vi "Read Strings from File.vi"(8 "Error In":errorcluster, 9 "Section Name":string, 11 "Path":path) -> (0 "Error Out":errorcluster, 1 "Found?":bool, 3 "Variant Database":variant)   [LabVIEW 2015]
doc: "This VI was created for use with the Read/Write Cluster VIs. It reads all the keys and their values from the specified section and puts them in two string arrays.\n\nFreeware from Moore Good Ideas, www.mooregoodideas.com. Do not remove this line."
uses:
  Suppress Error Code - Scalar.vi
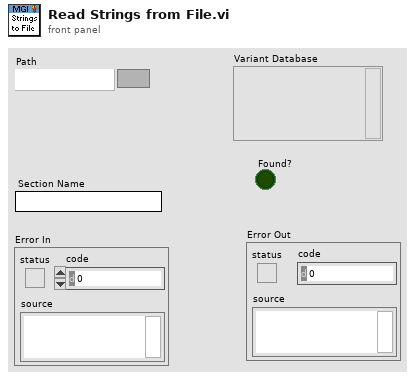
[diagram p1: front panel]
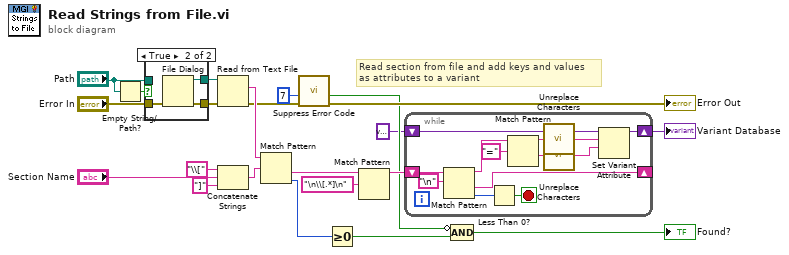
[diagram p0: block diagram]
diagram:
  # "Read section from file and add keys and values\nas attributes to a variant"
  n1 = Empty String/Path?(string/path="Path") -> (empty?=w2:bool)
  n2 = case shown="True" w2 {
    tunnel: "Error In" -> [w23 w27]
    tunnel: [w23 w26] -> w3
    tunnel: [w24 w25] -> w5
    tunnel: "Path" -> [w24 _]
    frame False {
    }
    frame True {
      n3 = File Dialog(8:w27) -> (0:w26:errorcluster, 3:w25:path)  [unwired: 8 out]
    }
  }
  n4 = Read from Text File(file (use dialog)=w5, error in=w3) -> (text=w18:string, error out=w14:errorcluster)  [unwired: 4 out]
  n5 = Concatenate Strings("\\[" ("string"), "Section Name", "]" ("string")) -> (w19:string)
  n6 = Match Pattern(string=w18, regular expression=w19) -> (after substring=w13:string, offset past match=w15:i32)  [unwired: 3 out]
  n7 = call-poly "Suppress Error Code.vi"("Error In"=w14, "Error Code"=7) -> ("Error Out"=→"Error Out":errorcluster, "Error Supressed?"=w9:bool)  [unwired: 8 out]
  n8 = Greater Or Equal To 0?(x=w15) -> (x >= 0?=w10:bool)
  n9 = Match Pattern(string=w13, regular expression="\n\\[.*]\n") -> (before substring=w16:string)  [unwired: 4 out]
  n10 = while {
    shift-right: [w38] -> _
    shift-left: w16 -> [w40]
    shift-right: [w33] -> w6
    shift-left: variant ("variant") -> [w34]
    stop <- w36 stop-if-true
    n11 = Match Pattern(string=w40, regular expression="\n") -> (before substring=w32:string, after substring=w38:string, offset past match=w37:i32)  [unwired: 2 out]
    n12 = Less Than 0?(x=w37) -> (x < 0?=w36:bool)
    n13 = Match Pattern(string=w32, regular expression="=") -> (before substring=w31:string, after substring=w30:string)  [unwired: 3 out]
    n14 = call "Unreplace Characters.vi"("String In"=w31) -> ("String Out"=w29:string)  [unwired: 1 out]
    n15 = call "Unreplace Characters.vi"("String In"=w30) -> ("String Out"=w28:string)  [unwired: 1 out]
    n16 = Set Variant Attribute(Variant=w34, name=w29, value=w28) -> (Variant out=w33:variant)  [unwired: 1 in, 2 out]
  }
  "Variant Database" <- w6
  n17 = Compound Arithmetic op=AND(invert w9, w10) -> (→"Found?":bool)
